vi "Parameterized.vi"() -> ()   [LabVIEW 2023]
doc: "This example inserts data into a table named parameterized in the LabVIEW.mdb database. The data is generated and inserted into the database once per second until you press the Stop button. \n\nThis VI uses a parameterized technique to insert data into the database. Since the SQL query can be parsed once and the data is \"filled in\" when needed, this results in a more efficient VI than if you used the Insert Data Into Database VI. However, the parameterized method is more difficult because it requires you to know more about SQL queries and data types."
uses:
  <vilib>/addons/database/Auxilliary.llb/DB Tools Parameter Info.ctl
  <vilib>/addons/database/Auxilliary.llb/DB Tools DataTypes.ctl
  <vilib>/addons/database/Auxilliary.llb/DB Tools Parameter Dir.ctl
  <vilib>/addons/database/Connection.llb/DB Tools Open Connec (Path).vi
  <vilib>/addons/database/Auxilliary.llb/DB Tools Format Datetime String (Time Stamp).vi
  <vilib>/addons/database/Command.llb/Cmd Set Parameter Value (C).vi
  <vilib>/addons/database/Command.llb/Cmd Execute.vi
  <vilib>/addons/database/Recordset.llb/Rec Destroy - Command.vi
  <vilib>/addons/database/Command.llb/Cmd Delete.vi
  <vilib>/addons/database/NI_Database_API.lvlib
panel:
  out "number of inserts":i32
  in  "Stop":bool
  in  "parameters":T1[](array[typedef])=[{"parameter name"="DAQ channel", "type"=enum."String", "direction"=enum."Input", "value"=variant}, {"parameter name"="", "type"=enum."Date/Time", "direction"=enum."Input", "value"=variant}, {"parameter name"="data", "type"=enum."Binary", "direction"=enum."Input", "value"=variant}]
  # "Overview: Demonstrates how to use a parameterized technique to insert data into a database.\nRequirements: Database Connectivity Toolkit\nInstructions:\n1. Run the VI. The parameter data is written to the database in a loop.\n2. Click Stop to stop the VI."
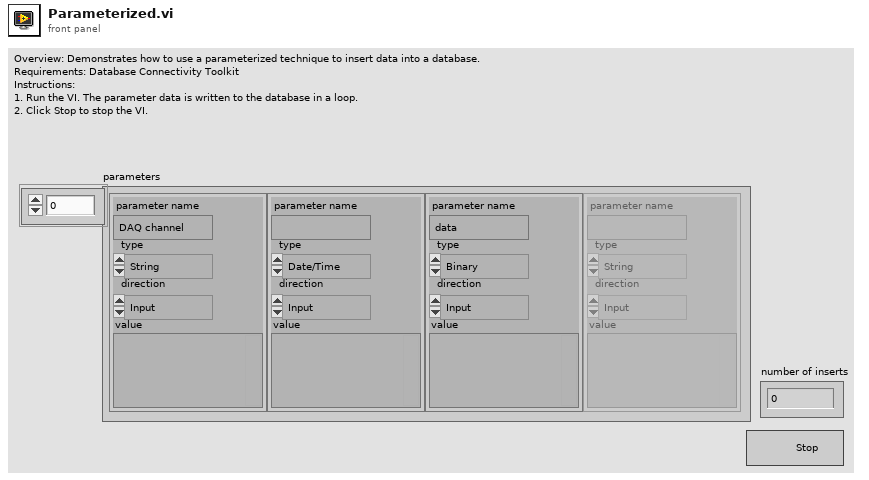
[diagram p1: front panel]
types:
  T1 = typedef "NI_Database_API.lvlib/DB Tools Parameter Info.ctl" = cluster{"parameter name":string, "type":T2, "direction":T3, "value":variant}
  T2 = typedef "NI_Database_API.lvlib/DB Tools DataTypes.ctl" = enum16{"String", "Long (I32)", "Single (SGL)", "Double (DBL)", "Date/Time", "Binary"}
  T3 = typedef "NI_Database_API.lvlib/DB Tools Parameter Dir.ctl" = enum32{"Input", "Output", "Input/Output", "Return Value"}
  T4 = typedef "NI_Database_API.lvlib/Conn ObjectReference.ctl" = refnum<k1>
  T5 = typedef "NI_Database_API.lvlib/Cmd ObjectReference.ctl" = refnum<k1>
  T6 = typedef "NI_Database_API.lvlib/Cmd-Rec Object Reference.ctl" = refnum<k1>
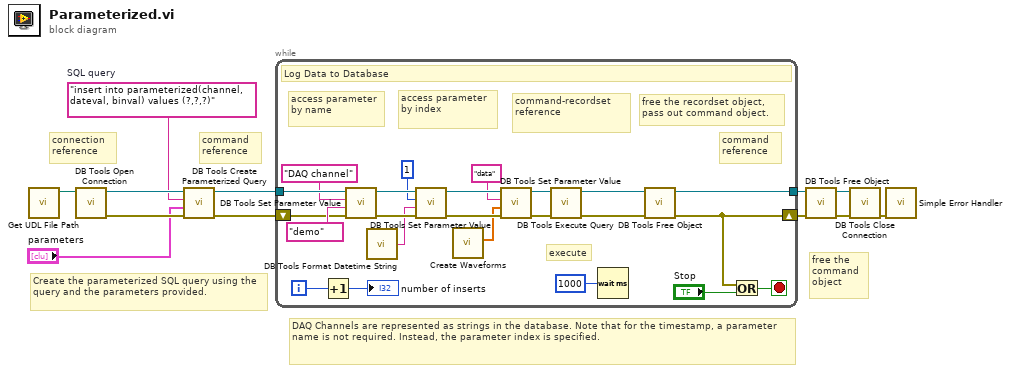
[diagram p0: block diagram]
diagram:
  w9 = "insert into parameterized(channel, dateval, binval) values (?,?,?)"  # SQL query
  # "DAQ Channels are represented as strings in the database. Note that for the timestamp, a parameter name is not required. Instead, the parameter index is specified."
  # "command \nreference"
  # "free the\ncommand\nobject"
  # "connection \nreference"
  # "Create the parameterized SQL query using the query and the parameters provided."
  n1 = call "Get UDL File Path.vi"() -> ("UDL file path"=w1:path)  [unwired: 11 in]
  n2 = call-poly <vilib>:"DB Tools Open Connection.vi"("connection information"=w1) -> ("error out"=w12:errorcluster, "connection reference"=w11:T4)  [unwired: 7 in]
  n3 = call <vilib>:"DB Tools Create Parameterized Query.vi"("error in (no error)"=w12, "parameters"="parameters", "SQL query"=w9, "connection reference"=w11) -> ("error out"=w7:errorcluster, "command reference"=w10:T5)  [unwired: 3 in, 1 out]
  n4 = while {
    tunnel: w10 -> [w35]
    shift-right: [w14] -> w5
    shift-left: w7 -> [w26]
    tunnel: [w16] -> w6
    i -> [w20]
    stop <- w22 stop-if-true
    # "free the recordset object, \npass out command object."
    # "execute"
    # "command \nreference"
    # "command-recordset reference"
    # "access parameter by index"
    # "access parameter by name"
    # "Log Data to Database"
    n5 = Increment(x=w20) -> (x+1=→"number of inserts":i32)
    n6 = call-poly <vilib>:"DB Tools Set Parameter Value.vi"("error in (no error)"=w26, "value"=tag "demo", "parameter index"="DAQ channel", "command reference"=w35) -> ("error out"=w34:errorcluster, "command reference out"=w33:T5)  [unwired: 4 in]
    n7 = call-poly <vilib>:"DB Tools Format Datetime String.vi"() -> ("date/time string"=w28:string)  [unwired: 1 in]
    n8 = call-poly <vilib>:"DB Tools Set Parameter Value.vi"("error in (no error)"=w34, "value"=w28, "parameter index"=1, "command reference"=w33) -> ("error out"=w32:errorcluster, "command reference out"=w31:T5)  [unwired: 4 in]
    n9 = call "Create Waveforms.vi"() -> ("core temperature"=w18:dbl[])  [unwired: 10 in, 1 out]
    n10 = call-poly <vilib>:"DB Tools Set Parameter Value.vi"("error in (no error)"=w32, "value"=w18, "parameter index"="data", "command reference"=w31) -> ("error out"=w25:errorcluster, "command reference out"=w24:T5)  [unwired: 4 in]
    n11 = call-poly <vilib>:"DB Tools Execute Query.vi"("error in (no error)"=w25, "command reference"=w24) -> ("error out"=w23:errorcluster, "command-recordset reference"=w17:T6)  [unwired: 6 in]
    n12 = Wait (ms)(milliseconds to wait=u32 1000) -> ()  [unwired: 1 out]
    n13 = call-poly <vilib>:"DB Tools Free Object.vi"("error in (no error)"=w23, "command-recordset reference"=w17) -> ("error out"=w14:errorcluster, "command reference"=w16:T5)  [unwired: 8 in]
    n14 = Or(x=w14, y="Stop") -> (x .or. y?=w22:bool)
  }
  n15 = call-poly <vilib>:"DB Tools Free Object.vi"("error in (no error)"=w5, "command reference"=w6) -> ("error out"=w4:errorcluster, "connection reference"=w3:T4)  [unwired: 8 in]
  n16 = call <vilib>:"DB Tools Close Connection.vi"("error in (no error)"=w4, "connection reference"=w3) -> ("error out"=w2:errorcluster)  [unwired: 5 in]
  n17 = call <vilib>:"Simple Error Handler.vi"("error in (no error)"=w2) -> ()  [unwired: 4 in, 5 out]
